vi "HV Load Test_production.vi"(5 "Published_Data_ID":string="HV39_", 7 "Reg0_State":string="State00", 10 "HV_Load_Steps_uA":dbl[](array[numeric])=[0.0, 5.0, 8.0, 10.0] format="%#_6p", 11 "Semiconductor Module Context":T1) -> (0 "error out":errorcluster)   [LabVIEW 2013]
uses:
  <vilib>/NI_TestStand_SemiconductorModule/NI_TestStand_Semiconductor_Module.lvlibp/PinMap/General/SemiconductorModuleContext.ctl
  <vilib>/NI_TestStand_SemiconductorModule/NI_TestStand_Semiconductor_Module.lvlibp/PinMap/DC Power/PinsToNIDCPowerSessions.vi
  <vilib>/NI_TestStand_SemiconductorModule/NI_TestStand_Semiconductor_Module.lvlibp/PinMap/Deprecated/PublishDataDoubleMultiplePinsMultipleInstruments.vi
  <vilib>/NI_TestStand_SemiconductorModule/NI_TestStand_Semiconductor_Module.lvlibp
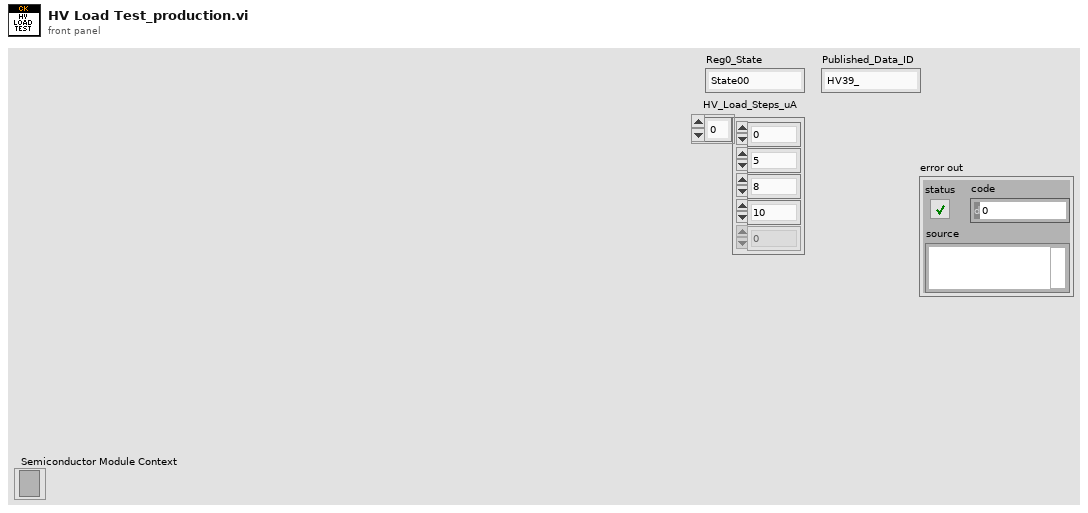
[diagram p1: front panel]
types:
  T1 = typedef "NI_TestStand_Semiconductor_Module.lvlibp/SemiconductorModuleContext.ctl" = refnum<k7>
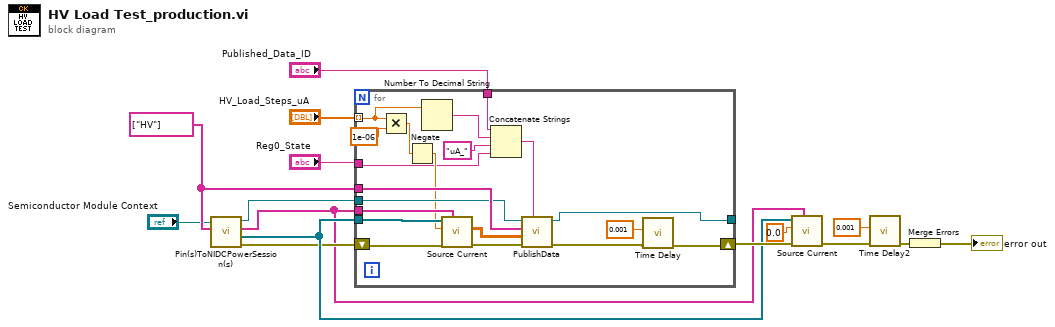
[diagram p0: block diagram]
diagram:
  w10 = string[] ["HV"] ("Pins")
  n1 = call-poly <vilib>:"Pin(s)ToNIDCPowerSession(s).vi"("Pins"=w10, "Semiconductor Module Context"="Semiconductor Module Context") -> ("error out"=w7:errorcluster, "Instrument Sessions"=w11:refnum<k15>[], "Channel Lists"=w6:string[], "Semiconductor Module Context Out"=w15:T1)  [unwired: 5 in, 1 out]
  n2 = for {
    tunnel: w10 -> [w34]
    tunnel: w15 -> [w32]
    tunnel: w6 -> [w27]
    tunnel: "HV_Load_Steps_uA" -> [w19] mode=indexing
    tunnel: w11 -> [w30]
    shift-right: [w18] -> w12
    shift-left: w7 -> [w31]
    tunnel: "Published_Data_ID" -> [w25]
    tunnel: [w24] -> _
    tunnel: "Reg0_State" -> [w20]
    n3 = Multiply(x=w19, y=1e-06) -> (x*y=w21:dbl)
    n4 = Negate(x=w21) -> (-x=w22:dbl)
    n5 = Number To Decimal String(number=w19) -> (decimal integer string=w29:string)  [unwired: 1 in]
    n6 = call "Source Current.vi"("Channel Lists"=w27, "error in (no error)"=w31, "current level"=w22, "Instrument Sessions In"=w30) -> ("error out"=w35:errorcluster, "voltage measurements"=w33:dbl[][])  [unwired: 4 in, 2 out]
    n7 = Concatenate Strings(w25, w29, "uA_" ("string"), w20) -> (w26:string)
    n8 = call-poly <vilib>:"PublishData.vi"("Measurement Id"=w26, "error in (no error)"=w35, "Data In"=w33, "Pins"=w34, "Semiconductor Module Context"=w32) -> ("error out"=w17:errorcluster, "Semiconductor Module Context Out"=w24:T1)  [unwired: 5 in]
    n9 = call "Time Delay"("error in (no error)"=w17, "Delay Time (s)"=0.001) -> ("error out"=w18:errorcluster)  [unwired: 9 in]
  }
  n10 = call "Source Current.vi"("Channel Lists"=w6, "error in (no error)"=w12, "current level"=0.0, "Instrument Sessions In"=w11) -> ("error out"=w3:errorcluster)  [unwired: 4 in, 3 out]
  n11 = call "Time Delay2"("error in (no error)"=w3, "Delay Time (s)"=0.001) -> ("error out"=w2:errorcluster)  [unwired: 9 in]
  n12 = Merge Errors(w2) -> (→"error out":errorcluster)
